vi "add_xml_headers.vi"(10 "xml":string, 11 "header string":string="<VariableSettings>\n") -> (3 "xml with headers":string)   [LabVIEW 2013]
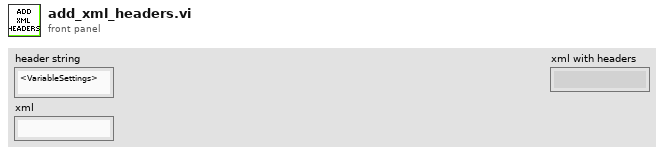
[diagram p1: front panel]
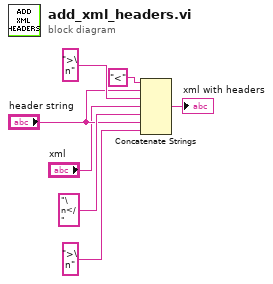
[diagram p0: block diagram]
diagram:
  n1 = Concatenate Strings("<" ("string"), "header string", ">\n" ("string"), "xml", "\n</" ("string"), "header string", ">\n" ("string")) -> (→"xml with headers":string)
